vi "Set Configuration.vi"(8 "error in (no error)":errorcluster, 10 "configuration":T1={"name"="Group", "direction"=enum."Tx", "cycle timing"={"priority"=100, "decimation"=1, "offset"=0}, "timeout behavior"=enum."Increment Late Count", "enable conversion"=FALSE}, 11 "Core Groups Configuration in":refnum<class "Group Configuration.lvclass">) -> (0 "error out":errorcluster, 3 "Core Groups Configuration out":refnum<class "Group Configuration.lvclass">)   [LabVIEW 2019, in "DSF Core.lvlib" / "Group Configuration.lvclass"]
uses:
  Group Configuration.lvclass
  Typedefs/Core Group Configuration.ctl
  Typedefs/DSF Direction.ctl
  Typedefs/DSF Timing Info.ctl
  Typedefs/DSF Timeout Behavior.ctl
  Group Configuration.lvclass/Group Configuration.ctl
  DSF Core.lvlib
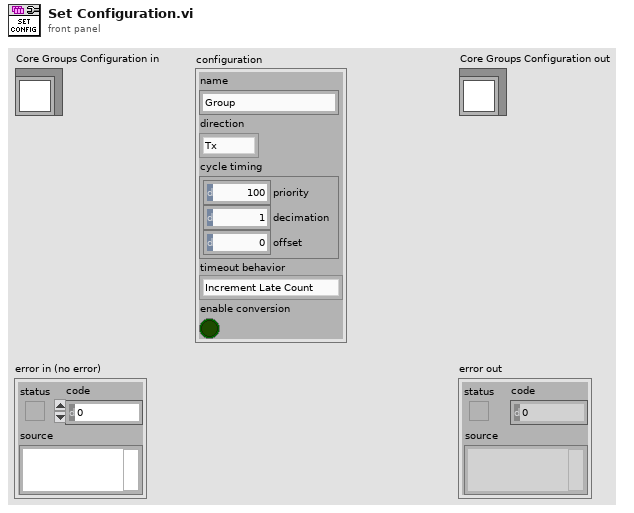
[diagram p1: front panel]
types:
  T1 = typedef "DSF Core.lvlib/Group Configuration.lvclass/Core Group Configuration.ctl" = cluster{"name":string, "direction":T2, "cycle timing":T3, "timeout behavior":T4, "enable conversion":bool}
  T2 = typedef "DSF Core.lvlib/DSF Direction.ctl" = enum8{"Tx", "Rx"}
  T3 = typedef "DSF Core.lvlib/DSF Timing Info.ctl" = cluster{"priority":u64, "decimation":u64, "offset":u64}
  T4 = typedef "DSF Core.lvlib/DSF Timeout Behavior.ctl" = enum8{"Increment Late Count", "Throw Error"}
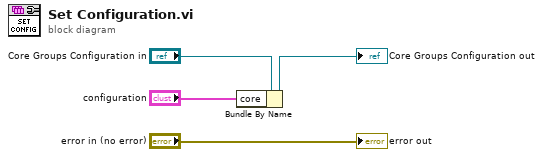
[diagram p0: block diagram]
diagram:
  n1 = Bundle By Name(cluster="Core Groups Configuration in", "core"="configuration") -> (→"Core Groups Configuration out":refnum<class "Group Configuration.lvclass">)
  "error out" <- "error in (no error)"
